vi "createError.vi"(7 "ErrorCode":T1, 11 "message":string) -> (0 "error out":errorcluster)   [LabVIEW 2011]
uses:
  Ctrls/EnumErrors.ctl
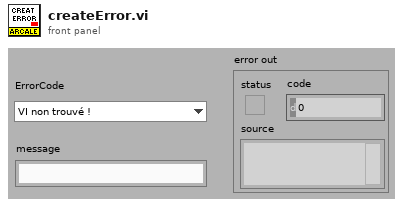
[diagram p1: front panel]
types:
  T1 = typedef "EnumErrors.ctl" = enum16{"VI non trouvé !", "Clé non trouvée", "Timeout", "Le VI tourne déjà", "Erreur de séparateur décimal", "Référence non trouvée"}
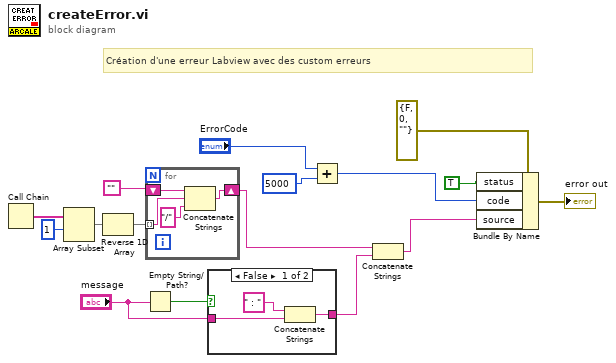
[diagram p0: block diagram]
diagram:
  # "Création d'une erreur Labview avec des custom erreurs"
  n1 = Call Chain() -> (call chain=w6:string[])
  n2 = Array Subset(array=w6, index=1) -> (w4:string[])  [unwired: 1 in]
  n3 = Reverse 1D Array(array=w4) -> (reversed array=w1:string[])
  n4 = Empty String/Path?(string/path="message") -> (empty?=w12:bool)
  n5 = for {
    tunnel: w1 -> [w18] mode=indexing
    shift-right: [w20] -> w2
    shift-left: "" -> [w19]
    n6 = Concatenate Strings(w19, w18, "/" ("string")) -> (w20:string)
  }
  n7 = case shown="False" w12 {
    tunnel: "message" -> [w22 w24]
    tunnel: [w23 w24] -> w10
    frame False {
      n8 = Concatenate Strings(" : " ("string"), w22) -> (w23:string)
    }
    frame True {
    }
  }
  n9 = Add(x="ErrorCode", y=5000) -> (x+y=w9:i32)
  n10 = Concatenate Strings(w2, w10) -> (w13:string)
  n11 = Bundle By Name(cluster=errorcluster {"status"=FALSE, "code"=0, "source"=""} ("error out"), "status"=TRUE, "code"=w9, "source"=w13) -> (→"error out":errorcluster)
